vi "DAQmx.Read.vi"(8 "error in":errorcluster, 11 "DAQmx in":refnum<class "DAQmx.lvclass">) -> (0 "error out":errorcluster, 2 "AIwfm":waveform(dbl)[](array[waveform]), 3 "DAQmx out":refnum<class "DAQmx.lvclass">, 4 "AI time (s)":dbl=2.0 format="%#_6p")   [LabVIEW 2019, in "DAQmx.lvclass"]
uses:
  DAQmx.lvclass
  DAQmx.lvclass/DAQmx.ctl
  <vilib>/DAQmx/read.llb/DAQmx Read (Analog 1D Wfm NChan NSamp).vi
  <vilib>/DAQmx/miscellaneous.llb/DAQmx Fill In Error Info.vi
  <resource>/objmgr/daqmx.rc
panel:
  out "AvailSampPerChan":u32[](array[numeric])
  in  "Show graph?":bool
  out "Waveform Graph":waveform(dbl)[](graph)
  out "P Check":bool[](array[boolean])
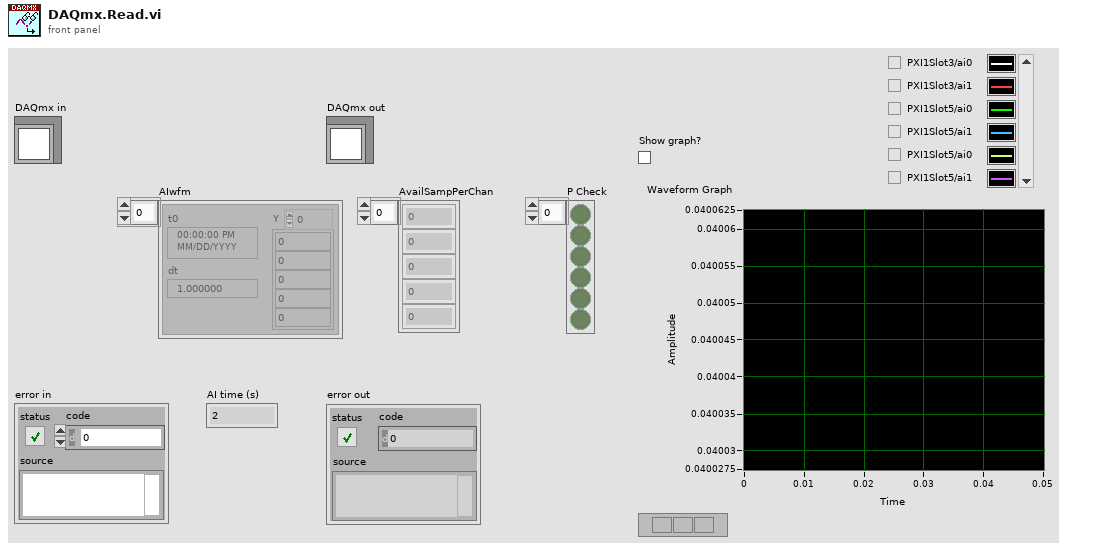
[diagram p1: front panel]
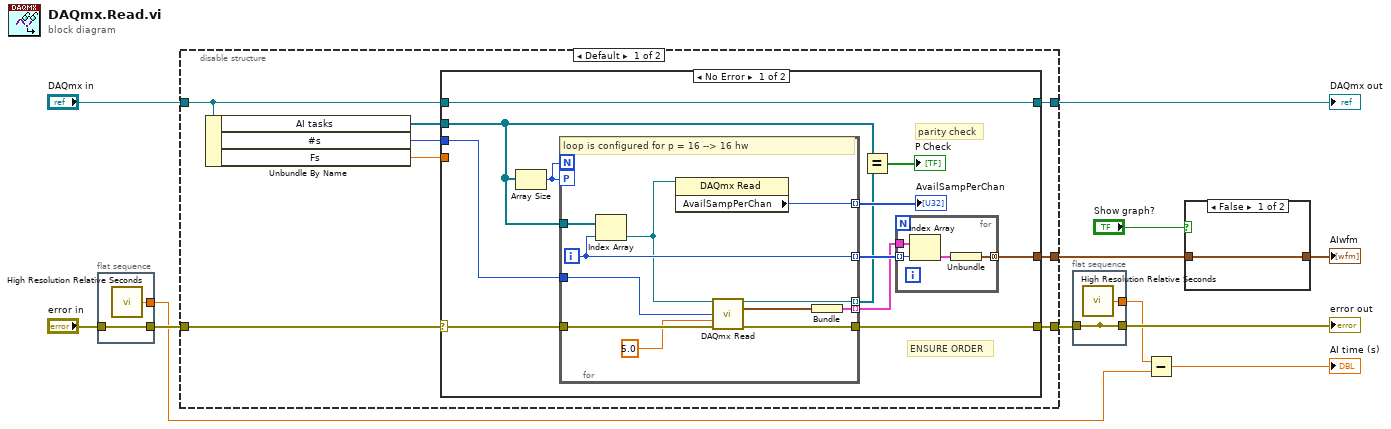
[diagram p0: block diagram]
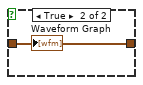
[diagram p4: hidden frame]
diagram:
  n1 = flat-sequence {
    tunnel: [w14] -> w6
    tunnel: "error in" -> [w14]
    tunnel: [w13] -> w5
    frame #0 {
      n2 = call <vilib>:"High Resolution Relative Seconds.vi"() -> ("relative seconds"=w13:dbl)
    }
  }
  n3 = disable-structure shown="Default" {
    disable-tunnel: [w21 w53] -> w4
    disable-tunnel: "DAQmx in" -> [w20 w52]
    disable-tunnel: w6 -> [w17 w53]
    disable-tunnel: [w19 w52] -> w8
    disable-tunnel: [w16 _] -> w9
    frame condition #0 (active) {
      n4 = Unbundle By Name(w20) -> ("AI tasks"=w18:refnum<k21>[], "#s"=w22:i32, "Fs"=w15:dbl)
      n5 = case shown="No Error" w17 {
        selector: w17 -> [w33 w51]
        tunnel: w22 -> [w23 _]
        tunnel: [w34 w51] -> w21
        tunnel: w18 -> [w32 _]
        tunnel: w20 -> [w31 w50]
        tunnel: [w31 w50] -> w19
        tunnel: w15 -> [_ _]
        tunnel: [w30 _] -> w16
        frame No Error {
          # "parity check"
          # "ENSURE ORDER"
          n6 = Array Size(array=w32) -> (size(s)=w27:i32)
          n7 = for {
            N: w27 -> [_]
            tunnel: w23 -> [w49]
            tunnel: [w46] -> w25 mode=indexing
            tunnel: w33 -> [w48]
            tunnel: [w47] -> w34
            tunnel: w32 -> [w45]
            workers-P: w27 -> [_]
            tunnel: [w44] -> w28 mode=indexing
            tunnel: [w43] -> w24 mode=indexing
            tunnel: [w40] -> w26 mode=indexing
            i -> [w44]
            # "loop is configured for p = 16 --> 16 hw"
            n8 = Index Array(array=w45, index=w44) -> (element=w41:refnum<k21>)
            n9 = property class="DAQmx Read"(reference=w41) -> ("AvailSampPerChan"=w40:u32)  [unwired: 1 in, 2 out]
            n10 = call-poly <vilib>:"DAQmx Read.vi"("task/channels in"=w41, "number of samples per channel"=w49, "timeout"=5.0, "error in"=w48) -> ("task out"=w43:refnum<k21>, "data"=w42:waveform(dbl)[], "error out"=w47:errorcluster)  [unwired: 9 in]
            n11 = Bundle("data"=w42) -> (w46:cluster{"data":waveform(dbl)[]})  [unwired: 1 in]
          }
          "AvailSampPerChan" <- w26
          n12 = Equal?(x=w32, y=w24) -> (x = y?=→"P Check":bool[])
          n13 = for {
            tunnel: w28 -> [w38] mode=indexing
            tunnel: w25 -> [w37]
            tunnel: [w36] -> w30 mode=concatenating
            n14 = Index Array(array=w37, index=w38) -> (element=w35:cluster{"data":waveform(dbl)[]})
            n15 = Unbundle(w35) -> ("data"=w36:waveform(dbl)[])
          }
        }
        frame Error {
        }
      }
    }
    frame condition #1 {
    }
  }
  "DAQmx out" <- w8
  n16 = flat-sequence {
    tunnel: w4 -> [w54]
    tunnel: [w54] -> _
    tunnel: [w55] -> w2
    tunnel: [w54] -> w3
    frame #0 {
      n17 = call <vilib>:"High Resolution Relative Seconds.vi"() -> ("relative seconds"=w55:dbl)
    }
  }
  n18 = Subtract(x=w2, y=w5) -> (x-y=→"AI time (s)":dbl)
  n19 = case shown="False" "Show graph?" {
    tunnel: w9 -> [w56 w57]
    tunnel: [w56 w57] -> w10
    frame False {
    }
    frame True {
      "Waveform Graph" <- w57
    }
  }
  "AIwfm" <- w10
  "error out" <- w3
